vi "Queued Temperature Controller Second Loop.vi"() -> ()   [LabVIEW 2013]
uses:
  Heater State.ctl
  <vilib>/Analysis/baseanly.llb/Mean (DBL).vi
  <vilib>/Analysis/NI_AALBase.lvlib
panel:
  in  "Stop Button":bool
  out "Current Temperature":dbl
  out "History":dbl(graph)
  in  "Temperature Control":dbl(slide)=1994.949494949495 scale=0.0..2500.0
  out "Heating Boolean":bool
  out "Mean":dbl format="%0.2f"
  out "Current Mean":dbl
  out "Min value":dbl
  out "Max value":dbl
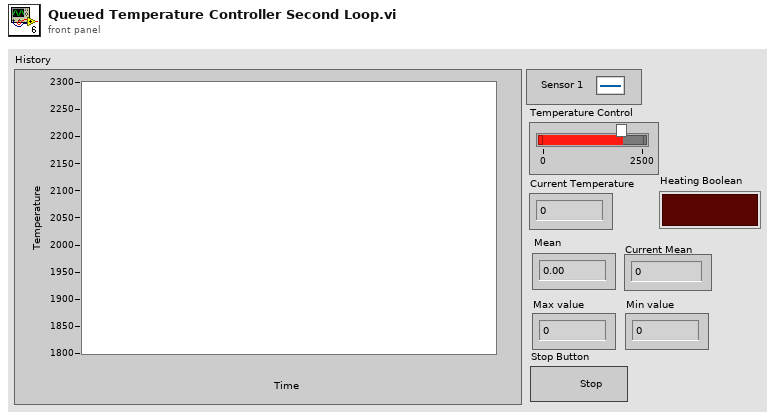
[diagram p1: front panel]
types:
  T1 = typedef "Heater State.ctl" = enum16{"Heat Off", "Heating", "Exit"}
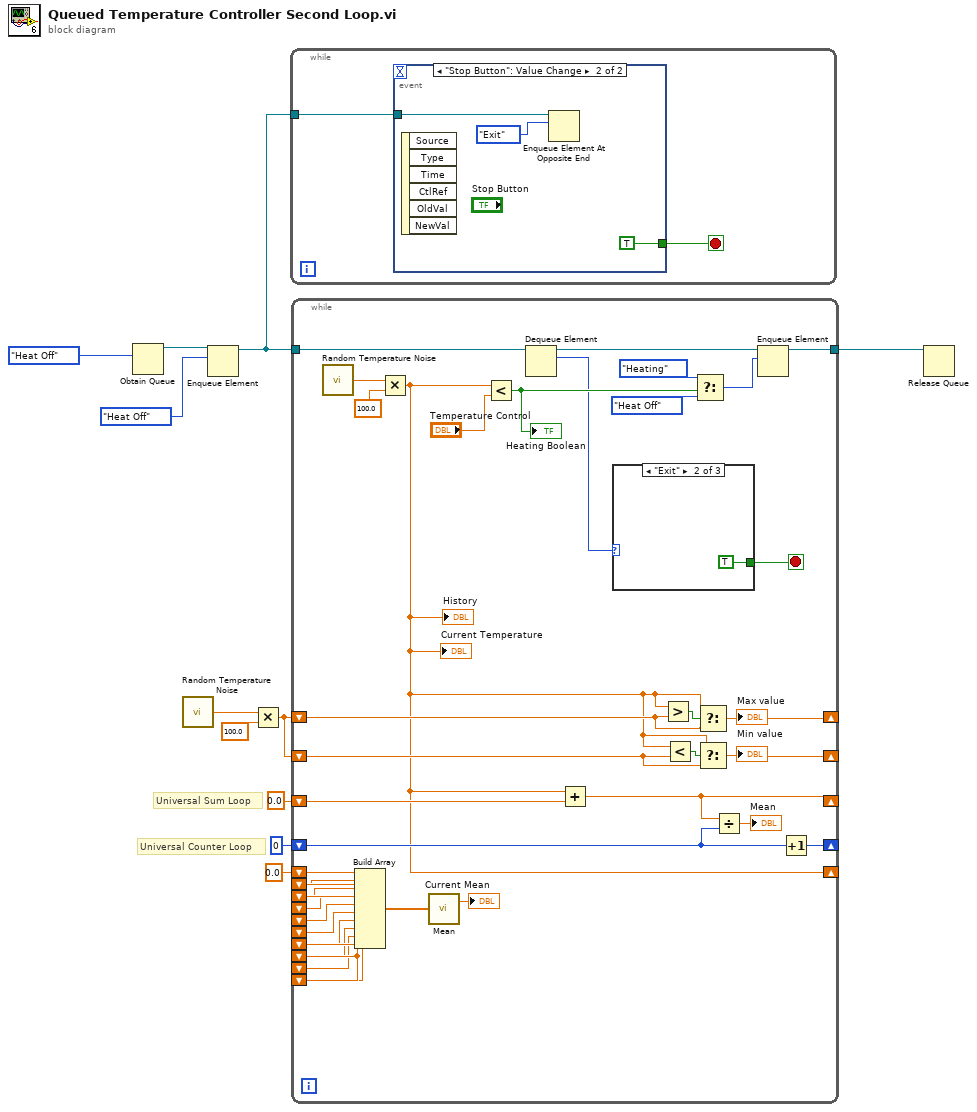
[diagram p0: block diagram]
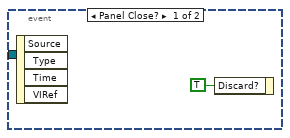
[diagram p2: hidden frame]
diagram:
  w6 = 0.0
  # "Universal Sum Loop"
  # "Universal Counter Loop"
  n1 = Obtain Queue(element data type=Heater_State."Heat Off" ("Heater State")) -> (queue out=w4:refnum<queue>)  [unwired: 4 in, 2 out]
  n2 = call "Random Temperature Noise.vi"() -> ("Temperature"=w10:dbl)  [unwired: 1 in]
  n3 = Enqueue Element(queue=w4, element=Heater_State."Heat Off" ("Heater State")) -> (queue out=w1:refnum<queue>)  [unwired: 2 in, 2 out]
  n4 = Multiply(x=w10, y=100.0) -> (x*y=w8:dbl)
  n5 = while {
    tunnel: w1 -> [w13]
    stop <- w12 stop-if-true
    n6 = event shown="[1] \"Stop Button\": Value Change" {
      selector: _ -> [_ _]
      dyn-events: _ -> [_ _]
      timeout: _ -> [_ _]
      tunnel: w13 -> [_ w16]
      tunnel: [_ TRUE] -> w12
      event Panel Close? {
        n7 = event-data() -> ()  [unwired: 1 in, 4 out]
        n8 = event-data("Discard?"=TRUE) -> ()  [unwired: 1 in, 1 out]
      }
      event "Stop Button": Value Change {
        n9 = event-data() -> ()  [unwired: 1 in, 6 out]
        n10 = Enqueue Element At Opposite End(queue=w16, element=Heater_State."Exit" ("Heater State")) -> ()  [unwired: 2 in, 3 out]
      }
    }
  }
  n11 = while {
    shift-right: [w33] -> _
    shift-left: 0.0 -> [w32]
    shift-right: [w49] -> _
    shift-left: w8 -> [w47]
    shift-right: [w48] -> _
    shift-left: w8 -> [w46]
    shift-right: [w20] -> _
    shift-left: w6 -> [w43]
    shift-left: w6 -> [w42]
    shift-left: w6 -> [w34]
    shift-left: w6 -> [w41]
    shift-left: w6 -> [w36]
    shift-left: w6 -> [w37]
    shift-right: [w44] -> _
    shift-left: 0 -> [w30]
    shift-left: w6 -> [w35]
    shift-left: w6 -> [w40]
    shift-left: w6 -> [w38]
    shift-left: w6 -> [w39]
    tunnel: w1 -> [w27]
    tunnel: [w22] -> w2
    stop <- w18 stop-if-true
    n12 = call "Random Temperature Noise.vi"() -> ("Temperature"=w52:dbl)  [unwired: 1 in]
    n13 = Build Array(w43, w42, w41, w40, w39, w38, w37, w36, w35, w34) -> (w28:dbl[])
    n14 = Multiply(x=w52, y=100.0) -> (x*y=w20:dbl)
    "History" <- w20
    "Current Temperature" <- w20
    n15 = call-poly <vilib>:"Mean.vi"("X"=w28) -> ("mean"=→"Current Mean":dbl)  [unwired: 1 out]
    n16 = Less?(x=w20, y="Temperature Control") -> (x < y?=w24:bool)
    "Heating Boolean" <- w24
    n17 = Dequeue Element(queue=w27) -> (queue out=w26:refnum<queue>, element=w19:T1)  [unwired: 2 in, 2 out]
    n18 = Add(x=w20, y=w32) -> (x+y=w33:dbl)
    n19 = case shown="\"Exit\"" w19 {
      tunnel: [_ TRUE _] -> w18
      frame "Heat Off" {
      }
      frame "Exit" {
      }
      frame "Heating" {
      }
    }
    n20 = Greater?(x=w20, y=w47) -> (0:w51:bool)
    n21 = Less?(x=w20, y=w46) -> (x < y?=w50:bool)
    n22 = Select(t=Heater_State."Heating" ("Heater State"), s=w24, f=Heater_State."Heat Off" ("Heater State")) -> (s? t:f=w23:T1)
    n23 = Select(t=w20, s=w51, f=w47) -> (s? t:f=w49:dbl)
    "Max value" <- w49
    n24 = Select(t=w20, s=w50, f=w46) -> (s? t:f=w48:dbl)
    "Min value" <- w48
    n25 = Divide(x=w33, y=w30) -> (x/y=→"Mean":dbl)
    n26 = Enqueue Element(queue=w26, element=w23) -> (queue out=w22:refnum<queue>)  [unwired: 2 in, 2 out]
    n27 = Increment(x=w30) -> (x+1=w44:i32)
  }
  n28 = Release Queue(queue=w2) -> ()  [unwired: 2 in, 3 out]
